vi "Listen.vi"(8 "error in (no error)":errorcluster, 11 "CIFTemplatePlugin in":refnum<class "CIFTemplatePlugin.lvclass">) -> (0 "error out":errorcluster, 3 "CIFTemplatePlugin out":refnum<class "CIFTemplatePlugin.lvclass">)   [LabVIEW 2021, in "CIFTemplatePlugin.lvclass"]
uses:
  CIFTemplatePlugin.lvclass
  D:/dev/CIF-LVCore/src/CIFCore/Class/CIFCorePlugin.lvclass
  CIFTemplatePlugin.lvclass/CIFTemplatePlugin.ctl
  CIFUtilities/CIFOutOfBand/CIFOutOfBand.lvclass/CIFOutOfBand.ctl
  CIFCore/Class/CIFCorePlugin.lvclass/CIFCorePlugin.ctl
  OOB/OOB_Rx/Receive/Check for OOB Commands.vi
  OOB/OOB_Rx/Receive/Read Data.vi
  OOB/OOB_Tx/Send/Update Data.vi
  CIFCore/Class/Accessors/Read Refresh.vi
  CIFUtilities/CIFOutOfBand/Read OOB DVR.vi
  OOB/OOB_Rx/Private/Command Settings.vi
  OOB/OOB_Rx/Private/Read Payload.vi
  CIFUtilities/CIFOutOfBand/Write OOB DVR.vi
  CIFUtilities/CIFOutOfBand/Utilities/Command to Bitwise Command.vi
  CIFUtilities/CIFOutOfBand/Accessors/Read Local OOB Data.vi
  CIFUtilities/CIFOutOfBand/Accessors/Write Local OOB Data.vi
  OOB/OOB_Rx/CIFTCustomOOB_Rx.lvclass
  D:/dev/CIF-LVCore/src/CIFUtilities/CIFOutOfBand/CIFOutOfBand.lvclass
  OOB/OOB_Tx/CIFCustomOOB_Tx.lvclass
  CIFCore/Class/CIFCorePlugin.lvclass
  CIFCore/Class/Typedef/Energized States.ctl
  D:/dev/CIF-LVCore/src/CIFTemplatePlugin/Class/CIFTemplatePlugin.lvclass
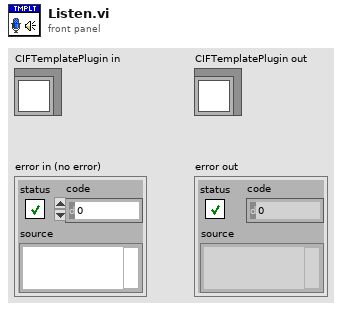
[diagram p1: front panel]
types:
  T1 = typedef "CIFCorePlugin.lvclass/Energized States.ctl" = enum16{"Listen", "Prepare", "Execute", "Housekeep", "Cleanup", "Destroy"}
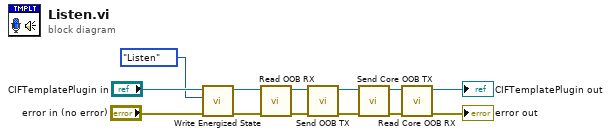
[diagram p0: block diagram]
diagram:
  n1 = call "Write Energized State.vi"("error in (no error)"="error in (no error)", "Energized State"=Energized_States."Listen", "CIFCorePlugin in"="CIFTemplatePlugin in") -> ("error out"=w8:errorcluster, "CIFCorePlugin out"=w9:refnum<class "CIFTemplatePlugin.lvclass">)  [unwired: 7 in]
  n2 = call "Read OOB RX.vi"("error in (no error)"=w8, "CIFTemplatePlugin in"=w9) -> ("error out"=w12:errorcluster, "CIFTemplatePlugin out"=w13:refnum<class "CIFTemplatePlugin.lvclass">)  [unwired: 8 in]
  n3 = call "Send OOB TX.vi"("error in (no error)"=w12, "CIFTemplatePlugin in"=w13) -> ("error out"=w4:errorcluster, "CIFTemplatePlugin out"=w5:refnum<class "CIFTemplatePlugin.lvclass">)  [unwired: 8 in]
  n4 = call "Send Core OOB TX.vi"("error in (no error)"=w4, "CIFCorePlugin in"=w5) -> ("error out"=w6:errorcluster, "CIFCorePlugin out"=w1:refnum<class "CIFTemplatePlugin.lvclass">)  [unwired: 8 in]
  n5 = call "Read Core OOB RX.vi"("error in (no error)"=w6, "CIFCorePlugin in"=w1) -> ("error out"=→"error out":errorcluster, "CIFCorePlugin out"=→"CIFTemplatePlugin out":refnum<class "CIFTemplatePlugin.lvclass">)  [unwired: 8 in]
